vi "Linear_fit_coefficientsph.vi"(1 "Template":path=path "/G4_2_HD/Users/paulhayden/Documents/Projects/Hong Roughness/XW data/XW_Corr.tpt") -> (2 "Saved Automatically?":bool, 3 "Tex Info String":string, 4 "Plot data file":path)   [LabVIEW 2018]
uses:
  Results_plotter_Global.vi
  Data plotting/subVIs/Plot_Values_Global.vi
  <vilib>/Analysis/NI_AALPro.lvlib
panel:
  out "intercept":dbl format="%.4f"
  out "slope":dbl format="%.4f"
  out "Current filename index":i32
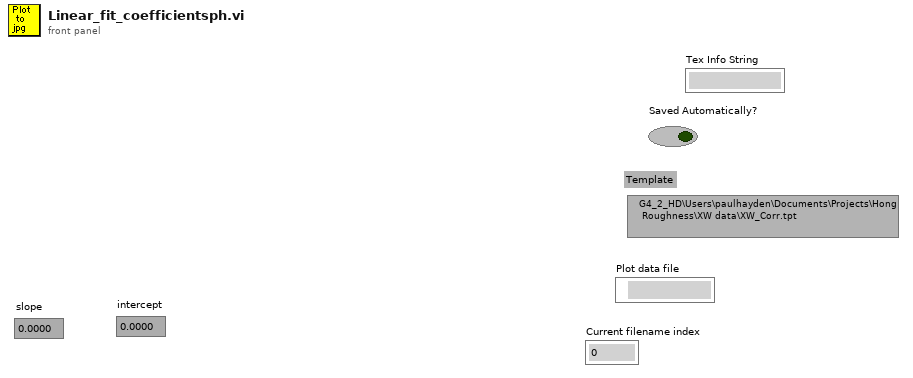
[diagram p1: front panel]
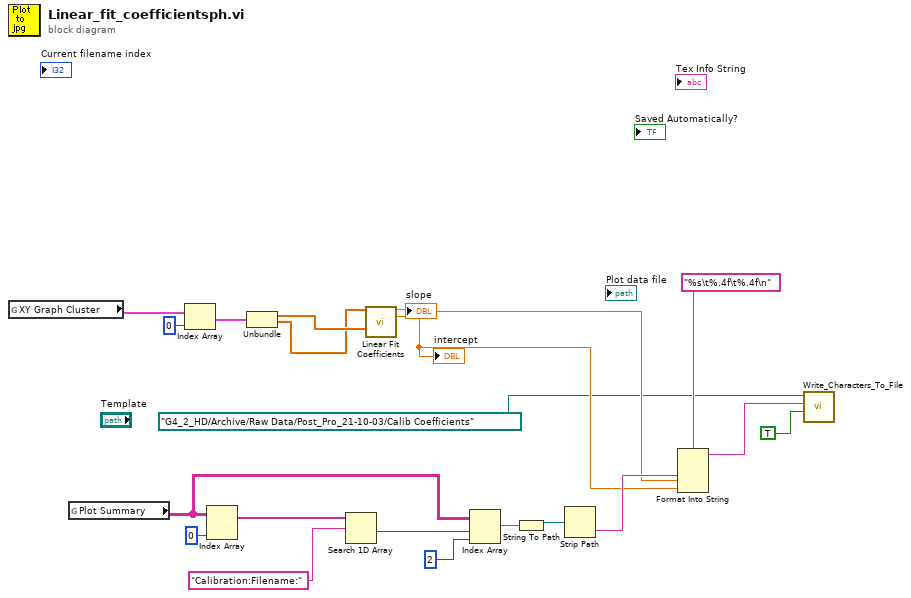
[diagram p0: block diagram]
diagram:
  n1 = global read "Plot_Values_Global.vi" "XY Graph Cluster"() -> (w1:cluster{dbl[], dbl[]}[])
  n2 = global read "Results_plotter_Global.vi" "Plot Summary"() -> (w13:string[][])
  n3 = Index Array(array=w1, index=0) -> (element=w19:cluster{dbl[], dbl[]})
  n4 = Index Array(array=w13, index (col)=0 ("disabled index (col)")) -> (element=w14:string[])  [unwired: 1 in]
  n5 = Unbundle(w19) -> (w18:dbl[], w17:dbl[])
  n6 = Search 1D Array(1D array=w14, element="Calibration:Filename:") -> (index of element=w12:i32)  [unwired: 1 in]
  n7 = call <vilib>:"Linear Fit Coefficients.vi"("Y"=w17, "X"=w18) -> ("slope"=w7:dbl, "intercept"=w6:dbl)  [unwired: 11 in, 1 out]
  "slope" <- w7
  "intercept" <- w6
  n8 = Index Array(array=w13, index (row)=w12, index (col)=2 ("disabled index (col)")) -> (element=w10:string)
  n9 = String To Path(string=w10) -> (path=w9:path)
  n10 = Strip Path(path=w9) -> (name=w8:string)  [unwired: 1 out]
  n11 = Format Into String(format string="%s\t%.4f\t%.4f\n", w8, w7, w6) -> (resulting string=w4:string)  [unwired: 2 in, 1 out]
  n12 = call "Write_Characters_To_File.vi"("file path (dialog if empty)"=path "/G4_2_HD/Archive/Raw Data/Post_Pro_21-10-03/Calib Coefficients" ("Output Filename"), "character string"=w4, "append to file? (new file:F)"=TRUE) -> ()  [unwired: 5 in, 1 out]
